vi "加V.vi"(3 "接收的AMI码":i8[](array[numeric])) -> (0 "索引值":u8[](array[numeric]), 1 "加+V和-V":i8[](array[numeric]))   [LabVIEW 2013]
panel:
  out "前一非0":i8
  in  "计连0":u8
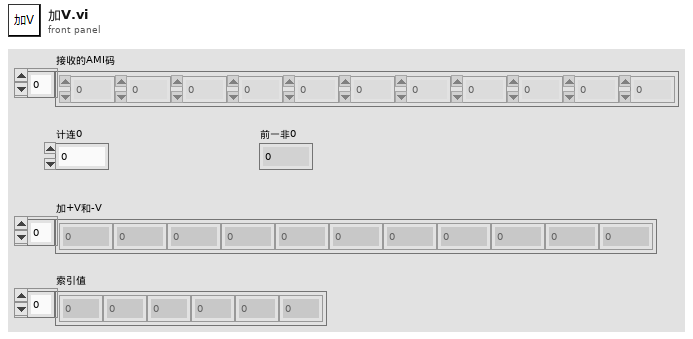
[diagram p1: front panel]
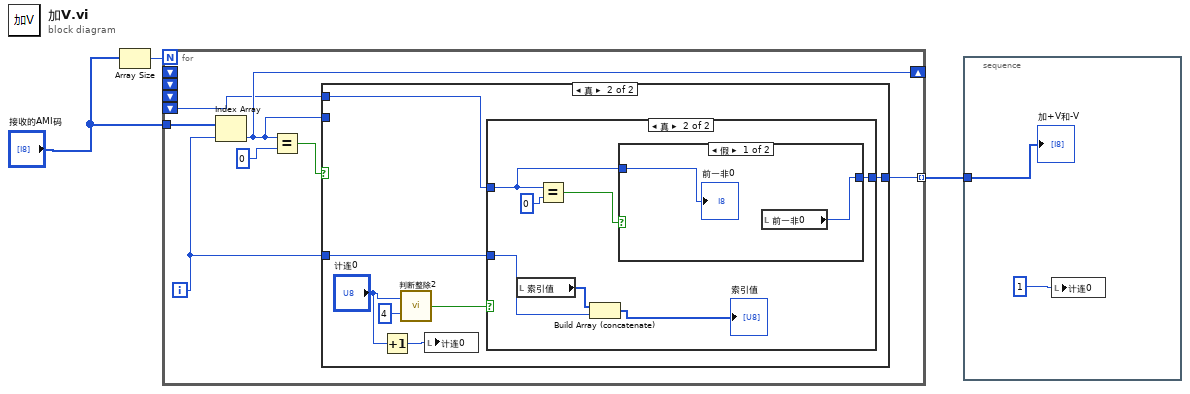
[diagram p0: block diagram]
diagram:
  n1 = Array Size(array="接收的AMI码") -> (size(s)=w3:i32)
  n2 = for {
    N: w3 -> [_]
    tunnel: "接收的AMI码" -> [w10]
    shift-right: [w5] -> _
    shift-left: _ -> [_]
    tunnel: [w7] -> w1 mode=indexing
    shift-left: _ -> [_]
    shift-left: _ -> [_]
    shift-left: _ -> [w4]
    i -> [w6]
    n3 = Index Array(array=w10, index=w6) -> (element=w5:i8)
    n4 = Equal?(x=w5, y=0) -> (x = y?=w8:bool)
    n5 = case shown="真" w8 {
      tunnel: [w11 w14] -> w7
      tunnel: w6 -> [_ w13]
      tunnel: w5 -> [w11 _]
      tunnel: w4 -> [_ w12]
      frame False {
      }
      frame True {
        n6 = Increment(x="计连0") -> (x+1=w17:u8)
        n7 = call "判断整除2.vi"("被除数"=4, "除数"="计连0") -> ("布尔 2"=w15:bool)
        n8 = local write "计连0"(w17) -> ()
        n9 = case shown="真" w15 {
          tunnel: w12 -> [_ w23]
          tunnel: [_ w22] -> w14
          tunnel: w13 -> [_ w21]
          frame False {
          }
          frame True {
            n10 = local read "索引值"() -> (w19:u8[])
            n11 = Equal?(x=w23, y=0) -> (x = y?=w24:bool)
            n12 = Build Array (concatenate)(w19, w21) -> (→"索引值":i32[])
            n13 = case shown="假" w24 {
              tunnel: w23 -> [w27 _]
              tunnel: [w26 _] -> w22
              frame False {
                n14 = local read "前一非0"() -> (w26:i8)
                "前一非0" <- w27
              }
              frame True {
              }
            }
          }
        }
      }
    }
  }
  n15 = stacked-sequence {
    tunnel: w1 -> [w29]
    frame #0 {
      n16 = local write "计连0"(1) -> ()
      "加+V和-V" <- w29
    }
  }
